vi "ESP301 Template.vi"   [LabVIEW 2015]
doc: "This block is for testing other ESP301 Blocks. Basically it became too annoying to haveto add the connect and disconnect blocks to everything especially if something is not supposed to be a standalone program."
panel:
  # "This is a good starter template for any program you are going to make for the esp 301"
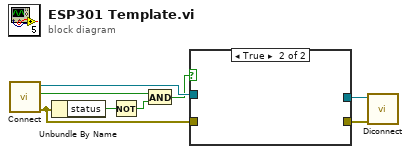
[diagram p0: block diagram]
diagram:
  n1 = call "Connect.vi"() -> ("error out"=w1:errorcluster, "Connected"=w4:bool, "VISA resource name out"=w8:refnum<visa-resource-name>)  [unwired: 5 in]
  n2 = Unbundle By Name(w1) -> ("status"=w5:bool)
  n3 = Not(x=w5) -> (.not. x?=w3:bool)
  n4 = And(x=w4, y=w3) -> (x .and. y?=w2:bool)
  n5 = case shown="True" w2 {
    tunnel: w8 -> [w10 _]
    tunnel: w1 -> [w9 _]
    tunnel: [w10 _] -> w7
    tunnel: [w9 _] -> w6
    frame False {
    }
    frame True {
    }
  }
  n6 = call "Diconnect.vi"("error in (no error)"=w6, "VISA resource name"=w7) -> ()  [unwired: 6 in]
